vi "TrackFinder Tester.vi"() -> ()   [LabVIEW 2013]
panel:
  out "Track Image":T1(plugin-control)
  out "error out":errorcluster
  in  "error in (no error)":errorcluster
  in  "AVI Path":path
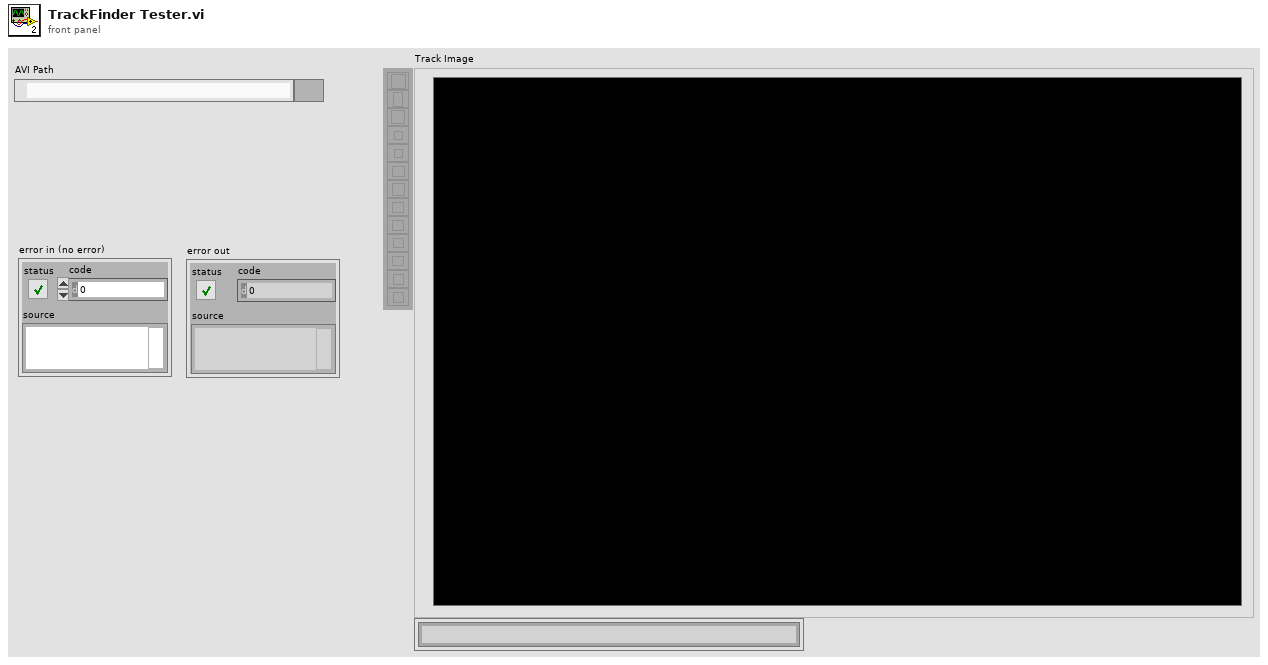
[diagram p1: front panel]
types:
  T1 = typedef "IMAQ Image.ctl" = refnum<image>
  T2 = typedef "IMAQ Line" = cluster{"Start X":i32, "Start Y":i32, "End X":i32, "End Y":i32}
  T3 = cluster{"Line":T2, "Score":dbl, "Straightness":dbl}[]
  T4 = typedef "ROI Descriptor" = cluster{"Global Rectangle":i32[], "Contours":cluster{"ID":enum32{"External", "Internal"}, "Type":u32, "Coordinates":i32[]}[]}
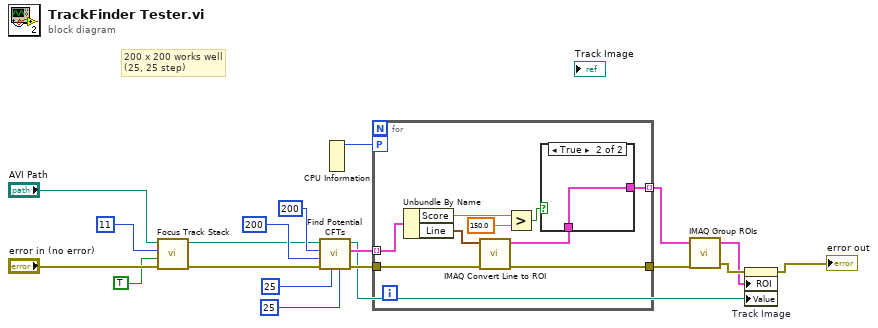
[diagram p0: block diagram]
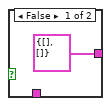
[diagram p2: hidden frame]
diagram:
  # "200 x 200 works well\n(25, 25 step)"
  n1 = call "Focus Track Stack.vi"("error in (no error)"="error in (no error)", "Grayscale?"=TRUE, "Kernel Size"=11, "Path"="AVI Path") -> ("error out"=w16:errorcluster, "Image"=w1:T1)  [unwired: 5 in, 1 out]
  n2 = call "Find Potential CFTs.vi"("dy"=25, "dx"=25, "error in (no error)"=w16, "ROI Height"=200, "ROI Width"=200, "Focused Image"=w1) -> ("error out"=w10:errorcluster, "Tracks"=w11:T3, "Focused Image out"=w8:T1)  [unwired: 3 in]
  n3 = CPU Information() -> (4:w3:i32)  [unwired: 3 out]
  n4 = for {
    tunnel: w11 -> [w28] mode=indexing
    tunnel: w10 -> [w26]
    tunnel: [w25] -> w9
    tunnel: [w20] -> w4 mode=indexing
    workers-P: w3 -> [_]
    n5 = Unbundle By Name(w28) -> ("Score"=w24:dbl, "Line"=w27:T2)
    n6 = call "IMAQ Convert Line to ROI"("error in (no error)"=w26, "Line"=w27) -> ("error out"=w25:errorcluster, "ROI Descriptor"=w22:T4)  [unwired: 7 in]
    n7 = Greater?(x=w24, y=150.0) -> (0:w21:bool)
    n8 = case shown="True" w21 {
      tunnel: w22 -> [_ w30]
      tunnel: [T4 {"Global Rectangle"=[], "Contours"=[]} ("ROI Descriptor") w30] -> w20
      frame False {
      }
      frame True {
      }
    }
  }
  n9 = call "IMAQ Group ROIs"("error in (no error)"=w9, "ROI Descriptors"=w4) -> ("error out"=w7:errorcluster, "ROI Descriptor out"=w5:T4)  [unwired: 2 in]
  n10 = property on="Track Image" class="ImageControl"(error in=w7, "ROI"=w5, "Value"=w8) -> (error out=→"error out":errorcluster)  [unwired: 1 in, 1 out]
